vi "extract_start.vi"(0 "multipart message in":string[](array[string]), 11 "error in (no error)":errorcluster) -> (4 "acq_length (ms)":dbl, 6 "bursts":string[](array[string]), 13 "Valid Message?":bool, 14 "Debug info":string, 15 "error out":errorcluster)   [LabVIEW 2019, in "mmW_commands.lvlib"]
doc: "- Extract_message (command specific)\no Validate parameters , JSON format and also command-specific parameters' formats and values\no Extract parameters from JSON to cluster (or directly to indicators\no Validate data field\no Extract data (if there is any…e.g at write_tx command)"
uses:
  mmW_commands.lvlib
  <vilib>/addons/_JKI.lib/Serialization/JSON/JKI JSON Serialization.lvlib
  typedefs/ports.ctl
  typedefs/mode.ctl
  typedefs/instr_hwclass.ctl
  typedefs/burst_mode.ctl
  Instrument Parameters.ctl
  TypeDefs/commands.ctl
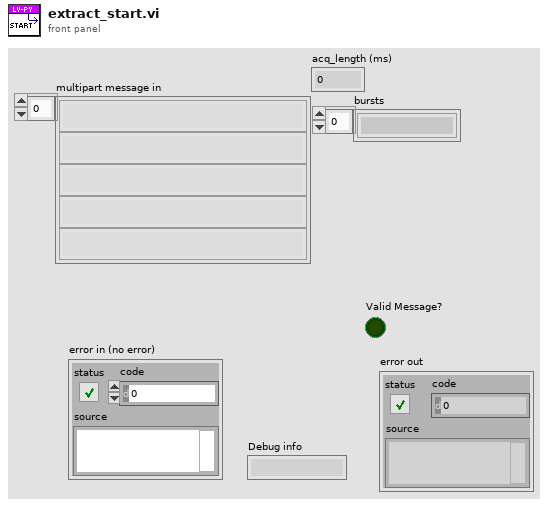
[diagram p1: front panel]
types:
  T1 = typedef "mmW_commands.lvlib/commands.ctl" = enum16{"configure_fs", "configure_rf", "configure_trigger", "equalization_enable", "equalization_start", "lo_sync_enable", "equalization_stop", "get_instrument_status", "get_versions", "initialize_hw", "pop_rx", "set_log_level", "Shutdown", "start", "start_instrument_app", "stop", "trans", "transceive", "trigger_burst", "trigger_sync_enable", "Write TX", "resp_generic", "resp_waveform", "send_trigger", "fetch", "transceive2"}
  T2 = typedef "mmW_commands.lvlib/Instrument Parameters.ctl" = cluster{"Write TX":cluster{"burstname":string, "burst_length":dbl}, "configure_fs":cluster{"port":T3, "fs":dbl}, "configure_rf":cluster{"port":T3, "fc":dbl, "gain":dbl}, "initialize_hw":cluster{"mode":T4, "hwclass":T5}, "start":cluster{"acq_length":dbl, "bursts":string[]}, "trigger_burst":cluster{"burst_mode":T6, "bursts":string[]}, "trigger_sync_enable":cluster{"Enable":bool}, "lo_sync_enable":cluster{"Enable":bool}, "equalization_enable":cluster{"Enable":bool}, "transceive":cluster{"burstname":string, "burst_mode":T6, "bursts":string[], "acq_length":dbl}, "generic_no_param":cluster{"no_param":string}}
  T3 = typedef "mmW_commands.lvlib/ports.ctl" = enum16{"rx", "tx"}
  T4 = typedef "mmW_commands.lvlib/mode.ctl" = enum16{"RF", "IF", "BB"}
  T5 = typedef "mmW_commands.lvlib/instr_hwclass.ctl" = enum16{"Simulated", "NI_mmW01", "Other"}
  T6 = typedef "mmW_commands.lvlib/burst_mode.ctl" = enum16{"burst", "continuous"}
  T7 = enum16{"big-endian, network order", "native, host order", "little-endian"}
  T8 = typedef "mmW_commands.lvlib/datatypes_.ctl" = enum16{"none", "string", "interleaved_I16", "interleaved_I32", "I16_array", "I32_array", "JSONstring"}
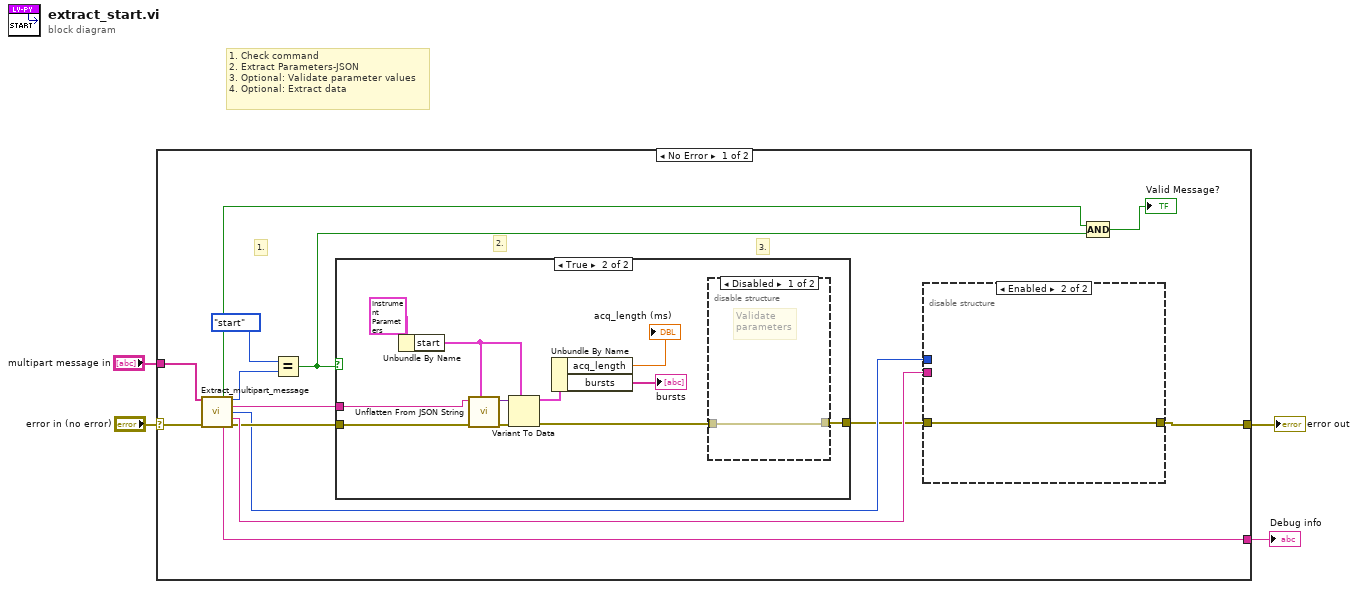
[diagram p0: block diagram]
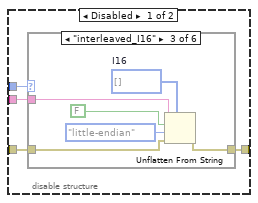
[diagram p4: hidden frame]
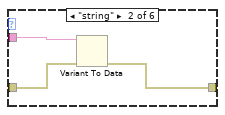
[diagram p6: hidden frame]
diagram:
  # "1. Check command\n2. Extract Parameters-JSON\n3. Optional: Validate parameter values\n4. Optional: Extract data"
  n1 = case shown="No Error" "error in (no error)" {
    selector: "error in (no error)" -> [w18 w50]
    tunnel: [w11 w50] -> w4
    tunnel: "multipart message in" -> [w13 _]
    tunnel: [w17 _] -> w1
    frame No Error {
      # "3."
      # "2."
      # "1."
      n2 = call "Extract_multipart_message.vi"("multipart message in"=w13, "error in (no error)"=w18) -> ("Valid message?"=w8:bool, "command out"=w10:T1, "parameters"=w16:string, "datatype"=w12:T8, "data out"=w15:string, "Debug info"=w17:string, "error out"=w14:errorcluster)  [unwired: 6 in, 1 out]
      n3 = Equal?(x=commands."start", y=w10) -> (x = y?=w7:bool)
      n4 = case shown="True" w7 {
        tunnel: w16 -> [_ w30]
        tunnel: w14 -> [w19 w27]
        tunnel: [w19 w22] -> w5
        frame False {
        }
        frame True {
          n5 = Unbundle By Name(T2 {"Write TX"={"burstname"="", "burst_length"=0.0}, "configure_fs"={"port"=enum."rx", "fs"=0.0}, "configure_rf"={"port"=enum."rx", "fc"=0.0, "gain"=0.0}, "initialize_hw"={"mode"=enum."RF", "hwclass"=enum."Simulated"}, "start"={"acq_length"=1000.0, "bursts"=[]}, "trigger_burst"={"burst_mode"=enum."burst", "bursts"=[]}, "trigger_sync_enable"={"Enable"=FALSE}, "lo_sync_enable"={"Enable"=FALSE}, "equalization_enable"={"Enable"=FALSE}, "transceive"={"burstname"="", "burst_mode"=enum."burst", "bursts"=[], "acq_length"=1000.0}, "generic_no_param"={"no_param"=""}} ("Instrument parameters")) -> ("start"=w25:cluster{"acq_length":dbl, "bursts":string[]})
          n6 = call <vilib>:"Unflatten From JSON String.vi"("Type and Defaults"=w25, "error in (no error)"=w27, "JSON String"=w30) -> ("error out"=w29:errorcluster, "Variant"=w28:variant)  [unwired: 7 in]
          n7 = Variant To Data(error in=w29, type=w25, Variant=w28) -> (data=w24:cluster{"acq_length":dbl, "bursts":string[]}, error out=w23:errorcluster)
          n8 = Unbundle By Name(w24) -> ("acq_length"=→"acq_length (ms)":dbl, "bursts"=→"bursts":string[])
          n9 = disable-structure shown="Disabled" {
            disable-tunnel: w23 -> [w31 _]
            disable-tunnel: [w31 _] -> w22
            frame Disabled {
              # "Validate \nparameters"
            }
            frame Enabled {
            }
          }
        }
      }
      n10 = disable-structure shown="Enabled" {
        disable-tunnel: w15 -> [w35 _]
        disable-tunnel: w5 -> [w34 w49]
        disable-tunnel: [w33 w49] -> w11
        disable-tunnel: w12 -> [w32 _]
        frame Disabled {
          n11 = case shown="\"interleaved_I16\"" w32 {
            tunnel: w35 -> [_ w39 w42 _ _ _]
            tunnel: w34 -> [w36 w38 w41 w46 w47 w48]
            tunnel: [w36 w37 w40 w46 w47 w48] -> w33
            frame "none", Default {
            }
            frame "string" {
              n12 = Variant To Data(error in=w38, Variant=w39) -> (error out=w37:errorcluster)  [unwired: 1 in, 1 out]
            }
            frame "interleaved_I16" {
              w45 = i16[] []  # I16
              n13 = Unflatten From String(type=w45, binary string=w42, data includes array or string size? (T)=FALSE, byte order (0:big-endian, network order)=T7."little-endian", error in (no error)=w41) -> (error out=w40:errorcluster)  [unwired: 2 out]
            }
            frame "interleaved_I32" {
            }
            frame "I16_array" {
            }
            frame "I32_array" {
            }
          }
        }
        frame Enabled {
        }
      }
      n14 = Compound Arithmetic op=AND(w8, w7) -> (→"Valid Message?":bool)
    }
    frame Error {
    }
  }
  "error out" <- w4
  "Debug info" <- w1
